vi "tab control.vi"() -> ()   [LabVIEW 2021]
panel:
  in  "a":dbl
  in  "tabcontrol":enum32{"page1", "page2"}(tab)
  in  "cluster":cluster{"b":dbl, "c":dbl}
  out "d":dbl
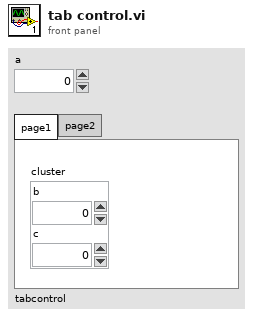
[diagram p1: front panel]
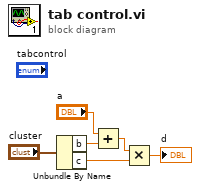
[diagram p0: block diagram]
diagram:
  n1 = Unbundle By Name("cluster") -> ("b"=w4:dbl, "c"=w2:dbl)
  n2 = Add(x="a", y=w4) -> (x+y=w3:dbl)
  n3 = Multiply(x=w3, y=w2) -> (x*y=→"d":dbl)
